vi "Eject.vi"(7 "Description":string, 8 "Command Info In":T1, 11 "Setpoint":dbl) -> (0 "Command Info Out":T1)   [LabVIEW 2017]
doc: "This template is useful for immediate subsystem actions that do not need deadband filtering\n\nBe sure to right-click and select New from Template and save with a new command name."
uses:
  <vilib>/Rock Robotics/WPI/Framework/Command Status Info.ctl
  <vilib>/Rock Robotics/WPI/Framework/Completion Status.ctl
  <vilib>/Rock Robotics/WPI/Framework/Completion Notifier.ctl
  Implementation/Intake Setpoints.ctl
  Implementation/Intake Operations.ctl
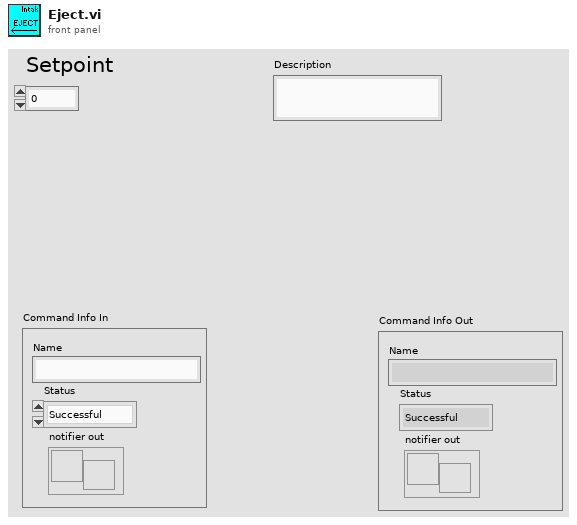
[diagram p1: front panel]
types:
  T1 = typedef "Command Status Info.ctl" = cluster{"Name":string, "Status":T2, "notifier out":T3}
  T2 = typedef "Completion Status.ctl" = enum16{"Successful", "Aborted", "Incomplete"}
  T3 = typedef "Completion Notifier.ctl" = refnum<notifier>
  T4 = typedef "Intake Setpoints.ctl" = cluster{"Operation":T5, "Setpoint":dbl, "Duration":dbl}
  T5 = typedef "Intake Operations.ctl" = enum16{"Reserve", "Read Current", "Immediate", "Intake", "Eject", "Stop"}
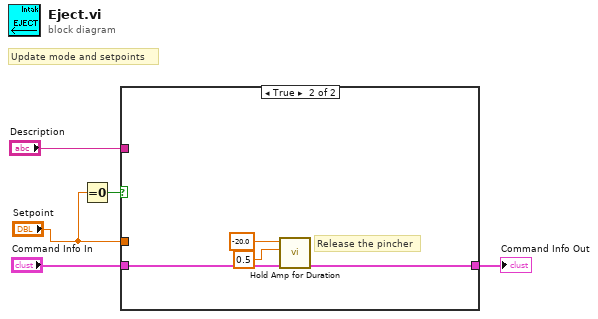
[diagram p0: block diagram]
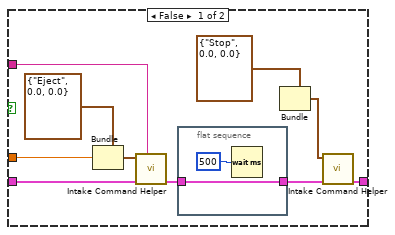
[diagram p2: hidden frame]
diagram:
  # "Update mode and setpoints"
  n1 = Equal To 0?(x="Setpoint") -> (x = 0?=w2:bool)
  n2 = case shown="True" w2 {
    tunnel: "Command Info In" -> [w15 w19]
    tunnel: "Description" -> [w14 _]
    tunnel: [w11 w18] -> w3
    tunnel: "Setpoint" -> [w6 _]
    frame False {
      n3 = Bundle(cluster=T4 {"Operation"=enum."Eject", "Setpoint"=0.0, "Duration"=0.0} ("SubSystem Data"), "Setpoint"=w6) -> (w12:T4)  [unwired: 2 in]
      n4 = call "Intake Command Helper.vi"("Description"=w14, "Command Info In"=w15, "SubSystem Data"=w12) -> ("Command Info Out"=w9:T1)  [unwired: 6 in, 2 out]
      n5 = flat-sequence {
        tunnel: [w16] -> w10
        tunnel: w9 -> [w16]
        frame #0 {
          n6 = Wait (ms)(milliseconds to wait=u32 500) -> ()  [unwired: 1 out]
        }
      }
      n7 = Bundle(cluster=T4 {"Operation"=enum."Stop", "Setpoint"=0.0, "Duration"=0.0} ("SubSystem Data")) -> (w7:T4)  [unwired: 3 in]
      n8 = call "Intake Command Helper.vi"("Command Info In"=w10, "SubSystem Data"=w7) -> ("Command Info Out"=w11:T1)  [unwired: 7 in, 2 out]
    }
    frame True {
      # "Release the pincher"
      n9 = call "Hold Amp for Duration.vi"("Command Info In"=w19, "Duration (s)"=0.5, "Setpoint"=-20.0) -> ("Command Info Out"=w18:T1)  [unwired: 8 in]
    }
  }
  "Command Info Out" <- w3
